vi "Project Point.vi"(10 "orientation (deg)":dbl, 11 "coordinates":dbl[](array[numeric])) -> (2 "projected point":cluster{"x":dbl, "y":dbl}, 3 "first point":cluster{"x":dbl, "y":dbl})   [LabVIEW 2020]
doc: "Use vertical value to determine which point is good and which needs to be recomputed.\nProject the original distance, but at the orientation angle instead of the Feret orientation.\n\nThis appears to be a pretty good approximation of diameter."
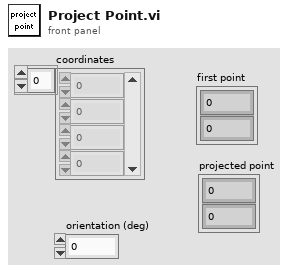
[diagram p1: front panel]
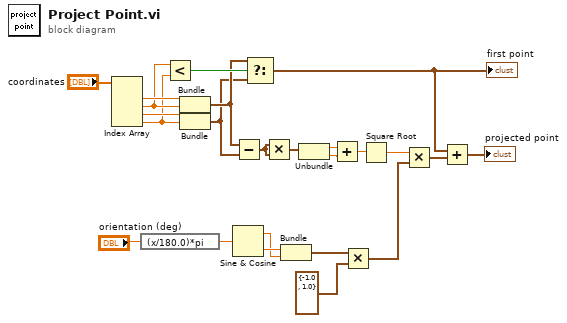
[diagram p0: block diagram]
diagram:
  n1 = Index Array(array="coordinates") -> (element #1=w15:dbl, element #2=w12:dbl, element #3=w14:dbl, element #4=w11:dbl)  [unwired: 4 in]
  n2 = expression code="(x/180.0)*pi" ("degrees to radians")("orientation (deg)") -> (w17:dbl)
  n3 = Less?(x=w12, y=w11) -> (x < y?=w10:bool)
  n4 = Bundle("Numeric"=w15, "Numeric"=w12) -> (w9:cluster{"Numeric":dbl, "Numeric":dbl})  [unwired: 1 in]
  n5 = Bundle("Numeric"=w14, "Numeric"=w11) -> (w8:cluster{"Numeric":dbl, "Numeric":dbl})  [unwired: 1 in]
  n6 = Sine & Cosine(0:w17) -> (1:w16:dbl, 2:w18:dbl)
  n7 = Subtract(x=w9, y=w8) -> (x-y=w19:cluster{"Numeric":dbl, "Numeric":dbl})
  n8 = Select(t=w9, s=w10, f=w8) -> (s? t:f=w6:cluster{"Numeric":dbl, "Numeric":dbl})
  "first point" <- w6
  n9 = Multiply(x=w19, y=w19) -> (x*y=w20:cluster{"Numeric":dbl, "Numeric":dbl})
  n10 = Bundle(w18, w16) -> (w2:cluster{dbl, dbl})  [unwired: 1 in]
  n11 = Unbundle(w20) -> ("Numeric"=w21:dbl, "Numeric"=w22:dbl)
  n12 = Add(x=w21, y=w22) -> (x+y=w23:dbl)
  n13 = Multiply(x=w2, y=cluster{dbl, dbl} {-1.0, 1.0} ("output cluster")) -> (x*y=w1:cluster{dbl, dbl})
  n14 = Square Root(x=w23) -> (sqrt(x)=w13:dbl)
  n15 = Multiply(x=w13, y=w1) -> (x*y=w7:cluster{dbl, dbl})
  n16 = Add(x=w6, y=w7) -> (x+y=→"projected point":cluster{dbl, dbl})
